vi "ImgData.vi"(1 "ImgNum":i16) -> (0 "Data":u8[][](array[numeric]))   [LabVIEW 2012]
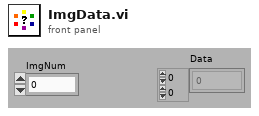
[diagram p1: front panel]
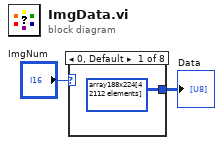
[diagram p0: block diagram]
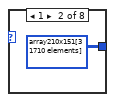
[diagram p2: hidden frame]
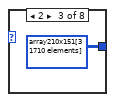
[diagram p3: hidden frame]
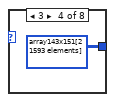
[diagram p4: hidden frame]
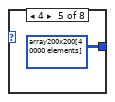
[diagram p5: hidden frame]
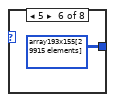
[diagram p6: hidden frame]
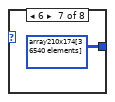
[diagram p7: hidden frame]
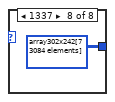
[diagram p8: hidden frame]
diagram:
  n1 = case shown="0, Default" "ImgNum" {
    tunnel: [u8[][] array188x224[42112 elements] ("data") u8[][] array210x151[31710 elements] ("data") u8[][] array210x151[31710 elements] ("data") u8[][] array143x151[21593 elements] ("data") u8[][] array200x200[40000 elements] ("data") u8[][] array193x155[29915 elements] ("data") u8[][] array210x174[36540 elements] ("data") u8[][] array302x242[73084 elements] ("data")] -> w2
    frame 0, Default {
    }
    frame 1 {
    }
    frame 2 {
    }
    frame 3 {
    }
    frame 4 {
    }
    frame 5 {
    }
    frame 6 {
    }
    frame 1337 {
    }
  }
  "Data" <- w2
